vi "子VI-查看某框.vi"(0 "输入框号（默认值0为整张图）":dbl format="%#_13g", 1 "框组":T3(array[cluster]), 2 "临界Z值":i32, 3 "反射图原始路径":path, 4 "临界面积百分比值":dbl, 5 "预先配置的灰度阈值":dbl, 6 "穿透图原始路径":path, 7 "部位信息":string[](array[string])=["", "34.500000", "32.500000", "1121", "34", "54.955926", "分层类", "不合格", ""], 12 "产品规格":cluster{"产品长度（周长）（mm）":dbl, "产品宽度（母线长）（mm）":dbl}) -> (14 "弥散类检测结果":string[][](table), 19 "分层类检测结果":string[][](table))   [LabVIEW 2018]
uses:
  <vilib>/vision/NI_Vision_Development_Module.lvlib
panel:
  in  "返回主界面":bool caption="辅助定性分析"
  in  "格式字符串 3":string="%f"
  in  "分隔符（'\\'代码显示） 2":string="\t"
  out "弥散和分层临界灰度值":i64
  out "弥散缺陷个数":i32
  out "分层缺陷个数":i32
  out "合格？ 弥散类":string="fencengThreshold"
  out "合格？分层类":string="fencengThreshold"
  in  "Tab Control":T1
  out "穿透ROI":T2(plugin-control)
  out "Threshold Image":T2(plugin-control)
  out "?":T2(plugin-control)
  out "?":T2(plugin-control)
  out "Threshold Image":T2(plugin-control)
  out "Threshold Image":T2(plugin-control)
  out "弥散测量结果":dbl[][](array[numeric]) format="%.2f"
  out "?":string
  out "面积 (pixels)":i32
  in  "格式字符串 2":string="%f"
  in  "分隔符（'\\'代码显示）":string="\t"
  out "分层测量结果":dbl[][](array[numeric]) format="%.2f"
  out "缺陷初步分类的临界值":sgl format="%#.3f"
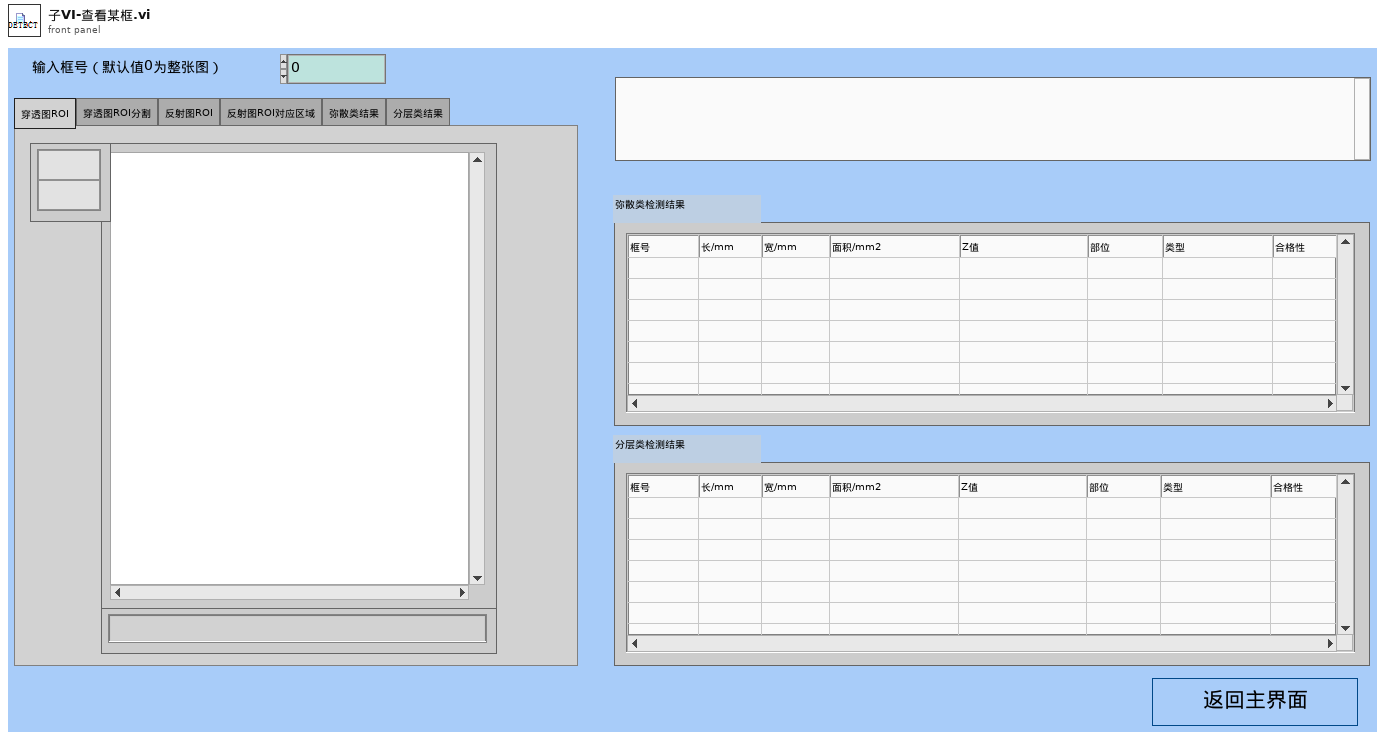
[diagram p1: front panel]
types:
  T1 = typedef "控件 1.ctl" = enum32{"穿透图ROI", "穿透图ROI分割", "反射图ROI", "反射图ROI对应区域", "弥散类结果", "分层类结果"}
  T2 = typedef "IMAQ Image.ctl" = refnum<image>
  T3 = cluster{"Global Rectangle":i32[], "Contours":cluster{"Contour Type":u32, "ROI Type":u32, "Points":i32[]}[]}[]
  T4 = cluster{"Zoom Tool":bool, "Selection Tool":bool, "Pan Tool":bool, "Point Tool":bool, "Line Tool":bool, "Rectangle Tool":bool, "Rotated Rectangle Tool":bool, "Polyline Tool":bool, "Polygon Tool":bool, "Freehand Tool":bool, "Closed Freehand Tool":bool, "Ellipse Tool":bool, "Annulus Tool":bool}
  T5 = typedef "Image Type" = u32
  T6 = typedef "Particle Parameters" = i32
  T7 = cluster{"Measurement Parameter":T6, "Range Lower Value":dbl, "Range Upper Value":dbl, "Range":bool, "Measurement Type":bool}[]
  T8 = cluster{"Global Rectangle":i32[], "Contours":cluster{"Contour Type":u32, "ROI Type":u32, "Points":i32[]}[]}
  T9 = cluster{"histogram":u32[], "Minimal Value":sgl, "Maximal Value":sgl, "Starting Value":sgl, "Interval Width":sgl, "Mean Value":sgl, "Standard  Variation":sgl, "Area (pixels)":i32}
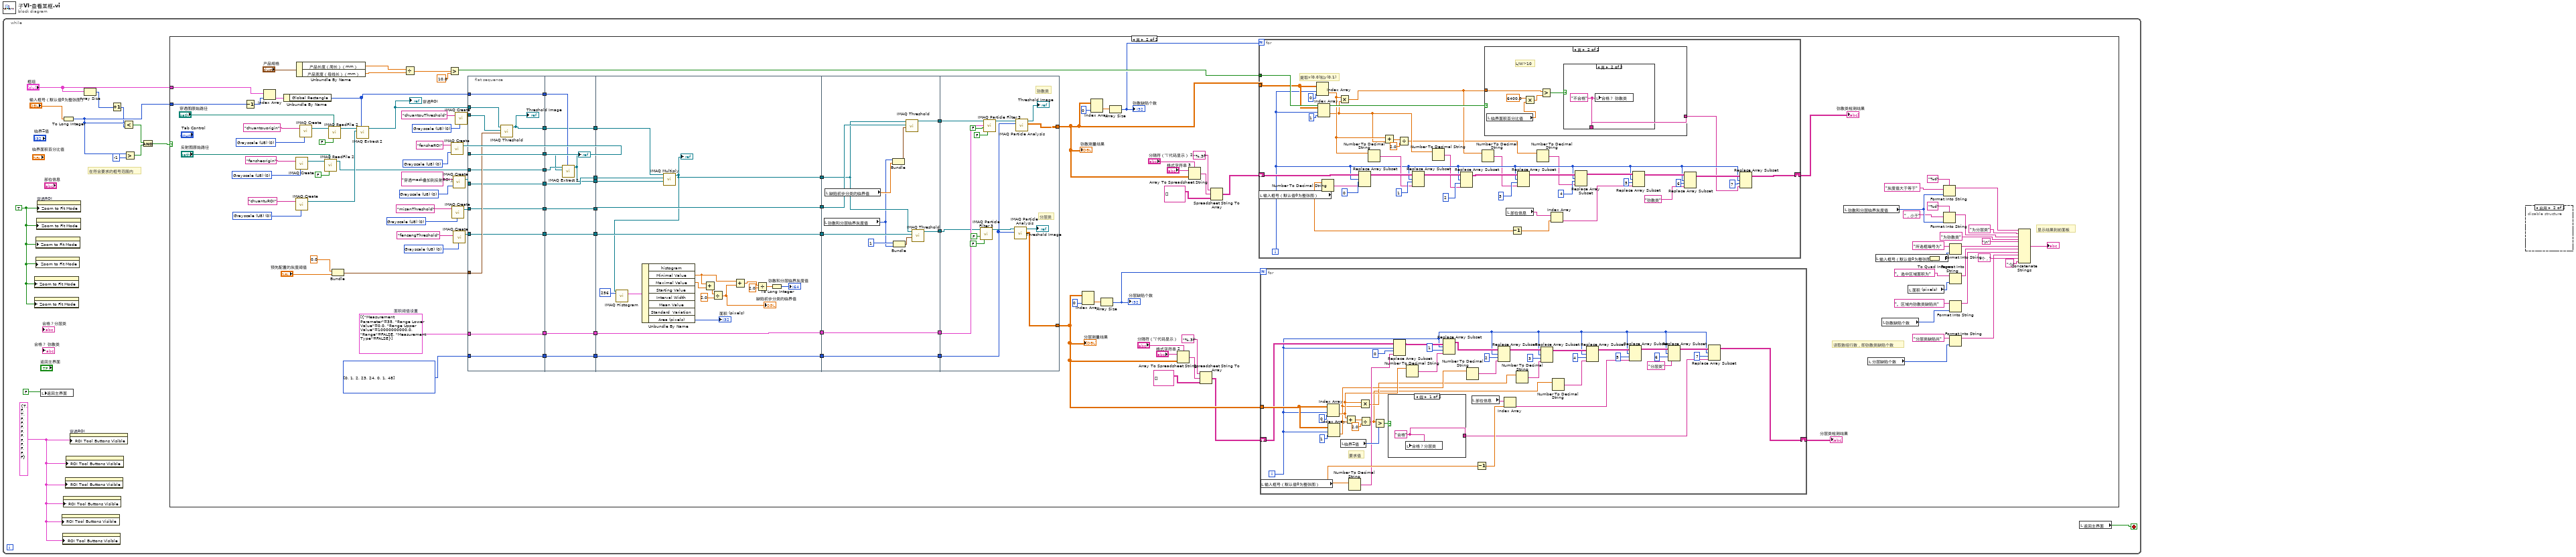
[diagram p0: block diagram]
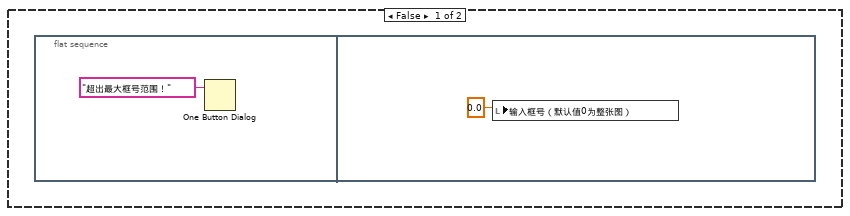
[diagram p2: hidden frame]
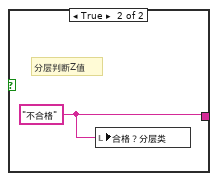
[diagram p3: hidden frame]
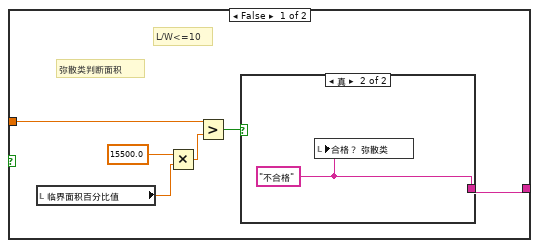
[diagram p4: hidden frame]
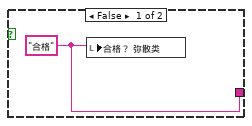
[diagram p5: hidden frame]
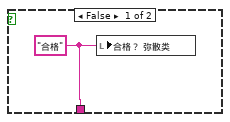
[diagram p6: hidden frame]
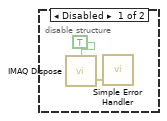
[diagram p7: hidden frame]
diagram:
  n1 = while {
    stop <- w5 stop-if-true
    w3 = T4 {"Zoom Tool"=TRUE, "Selection Tool"=FALSE, "Pan Tool"=TRUE, "Point Tool"=FALSE, "Line Tool"=FALSE, "Rectangle Tool"=FALSE, "Rotated Rectangle Tool"=FALSE, "Polyline Tool"=FALSE, "Polygon Tool"=FALSE, "Freehand Tool"=FALSE, "Closed Freehand Tool"=FALSE, "Ellipse Tool"=FALSE, "Annulus Tool"=FALSE} ("ROI Tool Buttons Visible:All Elements")
    w13 = TRUE ("Zoom to Fit Mode")
    # "在符合要求的框号范围内"
    n2 = property class="ImageControl"("Zoom to Fit Mode"=w13) -> ()  [unwired: 2 in, 2 out]
    n3 = property class="ImageControl"("Zoom to Fit Mode"=w13) -> ()  [unwired: 2 in, 2 out]
    n4 = property class="ImageControl"("Zoom to Fit Mode"=w13) -> ()  [unwired: 2 in, 2 out]
    n5 = property class="ImageControl"("Zoom to Fit Mode"=w13) -> ()  [unwired: 2 in, 2 out]
    n6 = property class="ImageControl"("Zoom to Fit Mode"=w13) -> ()  [unwired: 2 in, 2 out]
    n7 = property on="穿透ROI" class="ImageControl"("Zoom to Fit Mode"=w13) -> ()  [unwired: 2 in, 2 out]
    n8 = local write "返回主界面"(FALSE ("stop")) -> ()
    n9 = property class="ImageControl"("ROI Tool Buttons Visible"=w3) -> ()  [unwired: 2 in, 2 out]
    n10 = To Long Integer(number="输入框号（默认值0为整张图）") -> (32bit integer=w6:i32)
    n11 = property class="ImageControl"("ROI Tool Buttons Visible"=w3) -> ()  [unwired: 2 in, 2 out]
    n12 = property class="ImageControl"("ROI Tool Buttons Visible"=w3) -> ()  [unwired: 2 in, 2 out]
    n13 = property class="ImageControl"("ROI Tool Buttons Visible"=w3) -> ()  [unwired: 2 in, 2 out]
    n14 = property class="ImageControl"("ROI Tool Buttons Visible"=w3) -> ()  [unwired: 2 in, 2 out]
    n15 = property on="穿透ROI" class="ImageControl"("ROI Tool Buttons Visible"=w3) -> ()  [unwired: 2 in, 2 out]
    n16 = Array Size(array="框组") -> (size(s)=w2:i32)
    n17 = Increment(x=w2) -> (x+1=w1:i32)
    n18 = Less?(x=w6, y=w1) -> (x < y?=w11:bool)
    n19 = Greater?(x=w6, y=-1) -> (0:w10:bool)
    n20 = And(x=w11, y=w10) -> (x .and. y?=w4:bool)
    n21 = case shown="真" w4 {
      tunnel: "框组" -> [_ w17]
      tunnel: w6 -> [_ w16]
      frame False {
        n22 = flat-sequence {
          frame #0 {
            n23 = One Button Dialog(message="超出最大框号范围！" ("消息")) -> ()  [unwired: 1 in, 1 out]
          }
          frame #1 {
            n24 = local write "输入框号（默认值0为整张图）"(0.0 ("框号")) -> ()
          }
        }
      }
      frame True {
        w80 = T5 0 items=["Grayscale (U8)", "Grayscale (I16)", "Grayscale (SGL)", "Complex (CSG)", "RGB (U32)", "HSL (U32)", "RGB (U64)", "Grayscale (U16)"] ("Image Type")
        w81 = T5 0 items=["Grayscale (U8)", "Grayscale (I16)", "Grayscale (SGL)", "Complex (CSG)", "RGB (U32)", "HSL (U32)", "RGB (U64)", "Grayscale (U16)"] ("Image Type")
        w82 = T5 0 items=["Grayscale (U8)", "Grayscale (I16)", "Grayscale (SGL)", "Complex (CSG)", "RGB (U32)", "HSL (U32)", "RGB (U64)", "Grayscale (U16)"] ("Image Type")
        w86 = T5 0 items=["Grayscale (U8)", "Grayscale (I16)", "Grayscale (SGL)", "Complex (CSG)", "RGB (U32)", "HSL (U32)", "RGB (U64)", "Grayscale (U16)"] ("Image Type")
        w90 = T5 0 items=["Grayscale (U8)", "Grayscale (I16)", "Grayscale (SGL)", "Complex (CSG)", "RGB (U32)", "HSL (U32)", "RGB (U64)", "Grayscale (U16)"] ("Image Type")
        w64 = i32[] [0, 1, 2, 23, 24, 0, 1, 48] items=["Bounding Rect Width", "Bounding Rect Height", "Area"] ("Pixel Measurements")
        w65 = T7 [{"Measurement Parameter"=35, "Range Lower Value"=0.0, "Range Upper Value"=10000000000.0, "Range"=FALSE, "Measurement Type"=FALSE}]  # 面积阈值设置
        w101 = T5 0 items=["Grayscale (U8)", "Grayscale (I16)", "Grayscale (SGL)", "Complex (CSG)", "RGB (U32)", "HSL (U32)", "RGB (U64)", "Grayscale (U16)"] ("Image Type")
        w74 = T5 0 items=["Grayscale (U8)", "Grayscale (I16)", "Grayscale (SGL)", "Complex (CSG)", "RGB (U32)", "HSL (U32)", "RGB (U64)", "Grayscale (U16)"] ("Image Type")
        w105 = T5 0 items=["Grayscale (U8)", "Grayscale (I16)", "Grayscale (SGL)", "Complex (CSG)", "RGB (U32)", "HSL (U32)", "RGB (U64)", "Grayscale (U16)"] ("Image Type")
        # "显示结果到前面板"
        # "读取数组行数，即弥散类缺陷个数"
        n25 = Decrement(x=w16) -> (x-1=w107:i32)
        n26 = Index Array(array=w17, index=w107) -> (element=w108:T8)
        n27 = Unbundle By Name(w108) -> ("Global Rectangle"=w73:i32[])
        n28 = call "IMAQ Create"("Image Name"="fansheorigin", "Image Type"=w86) -> ("New Image"=w85:T2)  [unwired: 3 in, 1 out]
        n29 = call "IMAQ Create"("Image Name"="chuantuROI", "Image Type"=w90) -> ("New Image"=w89:T2)  [unwired: 3 in, 1 out]
        n30 = Unbundle By Name("产品规格") -> ("产品长度（周长）（mm）"=w96:dbl, "产品宽度（母线长）（mm）"=w95:dbl)
        n31 = call "IMAQ Create"("Image Name"="chuantouorigin", "Image Type"=w105) -> ("New Image"=w92:T2)  [unwired: 3 in, 1 out]
        n32 = call "IMAQ ReadFile 2"("Use File Path Image Type"=FALSE, "File Path"="反射图原始路径", "Image"=w85) -> ("Image Out"=w69:T2)  [unwired: 4 in, 4 out]
        n33 = call "IMAQ ReadFile 2"("Use File Path Image Type"=FALSE, "File Path"="穿透图原始路径", "Image"=w92) -> ("Image Out"=w93:T2)  [unwired: 4 in, 4 out]
        n34 = Bundle(0.0, "预先配置的灰度阈值"="预先配置的灰度阈值") -> (w63:cluster{dbl, "预先配置的灰度阈值":dbl})  [unwired: 1 in]
        n35 = call "IMAQ Extract 2"("Optional Rectangle"=w73, "Image Dst"=w89, "Image Src"=w93) -> ("Image Dst Out"=w71:T2)  [unwired: 7 in, 1 out]
        "穿透ROI" <- w71
        n36 = Divide(x=w96, y=w95) -> (x/y=w99:dbl)
        n37 = Greater?(x=w99, y=10.0) -> (0:w48:bool)
        n38 = call "IMAQ Create"("Image Name"="fansheROI", "Image Type"=w74) -> ("New Image"=w70:T2)  [unwired: 3 in, 1 out]
        n39 = call "IMAQ Create"("Image Name"="misanThreshold", "Image Type"=w80) -> ("New Image"=w67:T2)  [unwired: 3 in, 1 out]
        n40 = call "IMAQ Create"("Image Name"="穿透mask叠加到反射ROI上", "Image Type"=w101) -> ("New Image"=w68:T2)  [unwired: 3 in, 1 out]
        n41 = call "IMAQ Create"("Image Name"="fencengThreshold", "Image Type"=w81) -> ("New Image"=w66:T2)  [unwired: 3 in, 1 out]
        n42 = call "IMAQ Create"("Image Name"="chuantouThreshold", "Image Type"=w82) -> ("New Image"=w72:T2)  [unwired: 3 in, 1 out]
        n43 = flat-sequence {
          tunnel: w73 -> [w189]
          tunnel: w72 -> [w188]
          tunnel: w71 -> [w187]
          tunnel: w63 -> [w186]
          tunnel: w70 -> [w185]
          tunnel: w69 -> [w184]
          tunnel: [w189] -> w135
          tunnel: [w185] -> w134
          tunnel: [w184] -> w133
          tunnel: [w183] -> w132
          tunnel: w68 -> [w183]
          tunnel: [w182] -> w131
          tunnel: w67 -> [w181]
          tunnel: [w181] -> w130
          tunnel: [w180] -> w129
          tunnel: w66 -> [w180]
          tunnel: [w179] -> w128
          tunnel: w65 -> [w179]
          tunnel: [w178] -> w127
          tunnel: w64 -> [w178]
          tunnel: w135 -> [w199]
          tunnel: w134 -> [w190]
          tunnel: w133 -> [w191]
          tunnel: w132 -> [w198]
          tunnel: [w198] -> w126
          tunnel: [w197] -> w125
          tunnel: w131 -> [w197]
          tunnel: [w196] -> w124
          tunnel: w130 -> [w195]
          tunnel: [w195] -> w123
          tunnel: w129 -> [w194]
          tunnel: [w194] -> w122
          tunnel: w128 -> [w193]
          tunnel: [w193] -> w121
          tunnel: w127 -> [w192]
          tunnel: [w192] -> w120
          tunnel: w126 -> [w219]
          tunnel: w125 -> [w218]
          tunnel: w124 -> [w217]
          tunnel: [w216] -> w119
          tunnel: w123 -> [w216]
          tunnel: w122 -> [w215]
          tunnel: [w215] -> w118
          tunnel: [w210] -> w117
          tunnel: w121 -> [w209]
          tunnel: [w209] -> w116
          tunnel: w120 -> [w208]
          tunnel: [w208] -> w115
          tunnel: w119 -> [w231]
          tunnel: w118 -> [w230]
          tunnel: w117 -> [w229]
          tunnel: [w228] -> w114
          tunnel: [w227] -> w113
          tunnel: w116 -> [w226]
          tunnel: [w226] -> w112
          tunnel: w115 -> [w225]
          tunnel: [w225] -> w111
          tunnel: [w236] -> w45
          tunnel: [w240] -> w52
          tunnel: w114 -> [w233]
          tunnel: w113 -> [w232]
          tunnel: w112 -> [w238]
          tunnel: w111 -> [w237]
          frame #0 {
            n44 = call "IMAQ Threshold"("Range"=w186, "Image Dst"=w188, "Image Src"=w187) -> ("Image Dst Out"=w182:T2)  [unwired: 3 in, 5 out]
            "Threshold Image" <- w182
          }
          frame #1 {
            n45 = call "IMAQ Extract 2"("Optional Rectangle"=w199, "Image Dst"=w190, "Image Src"=w191) -> ("Image Dst Out"=w196:T2)  [unwired: 7 in, 1 out]
            "?" <- w196
          }
          frame #2 {
            n46 = call "IMAQ Multiply"("Image Src A"=w218, "Image Dst"=w219, "Image Src B"=w217) -> ("Image Dst Out"=w210:T2)  [unwired: 4 in, 1 out]
            "?" <- w210
            n47 = call "IMAQ Histogram"("Number of Classes"=256, "Image"=w210) -> ("Histogram Report"=w213:T9)  [unwired: 8 in, 1 out]
            n48 = Unbundle By Name(w213) -> ("Minimal Value"=w202:sgl, "Maximal Value"=w204:sgl, "Area (pixels)"=→"面积 (pixels)":i32)  [unwired: 5 out]
            n49 = Add(x=w202, y=w204) -> (x+y=w203:sgl)
            n50 = Divide(x=w203, y=sgl 2.0) -> (x/y=w201:sgl)
            "缺陷初步分类的临界值" <- w201
            n51 = Add(x=w202, y=w201) -> (x+y=w200:sgl)
            n52 = Divide(x=w200, y=sgl 2.0) -> (x/y=w205:sgl)
            n53 = To Long Integer(number=w205) -> (32bit integer=→"弥散和分层临界灰度值":i32)
          }
          frame #3 {
            n54 = local read "弥散和分层临界灰度值"() -> (w221:i64)
            n55 = local read "缺陷初步分类的临界值"() -> (w223:sgl)
            n56 = Bundle("弥散和分层临界灰度值"=w221, "缺陷初步分类的临界值"=w223) -> (w224:cluster{"弥散和分层临界灰度值":i64, "缺陷初步分类的临界值":sgl})  [unwired: 1 in]
            n57 = Bundle(1, "弥散和分层临界灰度值"=w221) -> (w220:cluster{i32, "弥散和分层临界灰度值":i64})  [unwired: 1 in]
            n58 = call "IMAQ Threshold"("Range"=w224, "Image Dst"=w231, "Image Src"=w229) -> ("Image Dst Out"=w227:T2)  [unwired: 3 in, 5 out]
            n59 = call "IMAQ Threshold"("Range"=w220, "Image Dst"=w230, "Image Src"=w229) -> ("Image Dst Out"=w228:T2)  [unwired: 3 in, 5 out]
          }
          frame #4 {
            # "分层类"
            # "弥散类"
            n60 = call "IMAQ Particle Filter 3"("Image Src"=w233, "Keep/Remove Particles (F)"=FALSE, "Reject Border? (F)"=FALSE) -> ("Image Dst Out"=w242:T2)  [unwired: 10 in, 2 out]
            n61 = call "IMAQ Particle Filter 3"("Image Src"=w232, "Selection Values"=w238, "Keep/Remove Particles (F)"=FALSE, "Reject Border? (F)"=FALSE) -> ("Image Dst Out"=w244:T2)  [unwired: 9 in, 2 out]
            n62 = call "IMAQ Particle Analysis"("Pixel Measurements"=w237, "Image"=w242) -> ("Particle Measurements (Pixels)"=w240:dbl[][], "Image Out (duplicate)"=→"Threshold Image":T2)  [unwired: 4 in, 4 out]
            n63 = call "IMAQ Particle Analysis"("Pixel Measurements"=w237, "Image"=w244) -> ("Particle Measurements (Pixels)"=w236:dbl[][], "Image Out (duplicate)"=→"Threshold Image":T2)  [unwired: 4 in, 4 out]
          }
        }
        n64 = Index Array(array=w52, index (col)=0 ("禁用的索引 (列)")) -> (element=w79:dbl[])  [unwired: 1 in]
        n65 = Index Array(array=w45, index (col)=0 ("禁用的索引 (列)")) -> (element=w77:dbl[])  [unwired: 1 in]
        n66 = Array Size(array=w79) -> (size(s)=w50:i32)
        "分层缺陷个数" <- w50
        n67 = Array Size(array=w77) -> (size(s)=w47:i32)
        "弥散缺陷个数" <- w47
        n68 = Array To Spreadsheet String(delimiter (Tab)="分隔符（'\\'代码显示）", array=w52, 3:"格式字符串 2") -> (spreadsheet string=w60:string)
        n69 = Array To Spreadsheet String(delimiter (Tab)="分隔符（'\\'代码显示） 2", array=w45, 3:"格式字符串 3") -> (spreadsheet string=w55:string)
        n70 = Spreadsheet String To Array(format string="%.3f", spreadsheet string=w60, array type (2D Dbl)=string[][] [] ("Array")) -> (array=w51:string[][])  [unwired: 1 in]
        n71 = Spreadsheet String To Array(format string="%.3f", spreadsheet string=w55, array type (2D Dbl)=string[][] [] ("Array")) -> (array=w46:string[][])  [unwired: 1 in]
        n72 = for {
          N: w47 -> [_]
          tunnel: w48 -> [w284]
          tunnel: w45 -> [w283]
          shift-right: [w263] -> w44
          shift-left: w46 -> [w271]
          i -> [w261]
          # "提取x(0,0)和y(0,1)"
          n73 = local read "输入框号（默认值0为整张图）"() -> (w249:dbl)
          n74 = Index Array(array=w283, index (row)=w261, index (col)=0 ("禁用的索引 (列)")) -> (element=w255:dbl)
          n75 = Index Array(array=w283, index (row)=w261, index (col)=1 ("禁用的索引 (列)")) -> (element=w254:dbl)
          n76 = Number To Decimal String(number=w249) -> (decimal integer string=w272:string)  [unwired: 1 in]
          n77 = Multiply(x=w255, y=w254) -> (x*y=w259:dbl)
          n78 = Replace Array Subset(array=w271, new element=w272, index (row)=w261, index (col)=0 ("索引 (列)")) -> (w270:string[][])
          n79 = Number To Decimal String(number=w255) -> (decimal integer string=w262:string)  [unwired: 1 in]
          n80 = Add(x=w255, y=w254) -> (x+y=w257:dbl)
          n81 = Divide(x=w257, y=2.0) -> (x/y=w253:dbl)
          n82 = Replace Array Subset(array=w270, new element=w262, index (row)=w261, index (col)=1 ("索引 (列)")) -> (w269:string[][])
          n83 = Number To Decimal String(number=w254) -> (decimal integer string=w260:string)  [unwired: 1 in]
          n84 = Replace Array Subset(array=w269, new element=w260, index (row)=w261, index (col)=2 ("索引 (列)")) -> (w268:string[][])
          n85 = Number To Decimal String(number=w259) -> (decimal integer string=w258:string)  [unwired: 1 in]
          n86 = case shown="真" w284 {
            tunnel: w259 -> [w290 w298]
            tunnel: [w288 w296] -> w246
            frame False {
              # "弥散类判断面积"
              # "L/W<=10"
              n87 = local read "临界面积百分比值"() -> (w286:dbl)
              n88 = Multiply(x=15500.0, y=w286) -> (x*y=w285:dbl)
              n89 = Greater?(x=w290, y=w285) -> (0:w289:bool)
              n90 = case shown="真" w289 {
                tunnel: [w291 w292] -> w288
                frame False {
                  w291 = "合格" ("合格？")
                  n91 = local write "合格？ 弥散类"(w291) -> ()
                }
                frame True {
                  w292 = "不合格" ("合格？")
                  n92 = local write "合格？ 弥散类"(w292) -> ()
                }
              }
            }
            frame True {
              # "L/W>10"
              n93 = local read "临界面积百分比值"() -> (w293:dbl)
              n94 = Multiply(x=6400.0, y=w293) -> (x*y=w295:dbl)
              n95 = Greater?(x=w298, y=w295) -> (0:w297:bool)
              n96 = case shown="真" w297 {
                tunnel: [w299 w300] -> w296
                frame False {
                  w299 = "合格" ("合格？")
                  n97 = local write "合格？ 弥散类"(w299) -> ()
                }
                frame True {
                  w300 = "不合格" ("合格？")
                  n98 = local write "合格？ 弥散类"(w300) -> ()
                }
              }
            }
          }
          n99 = local read "部位信息"() -> (w251:string[])
          n100 = Decrement(x=w249) -> (x-1=w250:dbl)
          n101 = Replace Array Subset(array=w268, new element=w258, index (row)=w261, index (col)=3 ("索引 (列)")) -> (w267:string[][])
          n102 = Number To Decimal String(number=w253) -> (decimal integer string=w252:string)  [unwired: 1 in]
          n103 = Index Array(array=w251, index=w250) -> (element=w248:string)
          n104 = Replace Array Subset(array=w267, new element=w252, index (row)=w261, index (col)=4 ("索引 (列)")) -> (w266:string[][])
          n105 = Replace Array Subset(array=w266, new element=w248, index (row)=w261, index (col)=5 ("索引 (列)")) -> (w265:string[][])
          n106 = Replace Array Subset(array=w265, new element="弥散类" ("新元素/子数组"), index (row)=w261, index (col)=6 ("索引 (列)")) -> (w264:string[][])
          n107 = Replace Array Subset(array=w264, new element=w246, index (row)=w261, index (col)=7 ("索引 (列)")) -> (w263:string[][])
        }
        "弥散类检测结果" <- w44
        n108 = for {
          N: w50 -> [_]
          tunnel: w52 -> [w167]
          shift-right: [w145] -> w49
          shift-left: w51 -> [w156]
          i -> [w140]
          # "要求值"
          n109 = local read "输入框号（默认值0为整张图）"() -> (w165:dbl)
          n110 = Index Array(array=w167, index (row)=w140, index (col)=0 ("禁用的索引 (列)")) -> (element=w144:dbl)
          n111 = Index Array(array=w167, index (row)=w140, index (col)=1 ("禁用的索引 (列)")) -> (element=w143:dbl)
          n112 = local read "临界Z值"() -> (w173:i32)
          n113 = Add(x=w144, y=w143) -> (x+y=w174:dbl)
          n114 = Number To Decimal String(number=w165) -> (decimal integer string=w157:string)  [unwired: 1 in]
          n115 = Multiply(x=w144, y=w143) -> (x*y=w142:dbl)
          n116 = Divide(x=w174, y=2.0) -> (x/y=w139:dbl)
          n117 = Greater?(x=w139, y=w173) -> (0:w175:bool)
          n118 = case shown="假" w175 {
            tunnel: [w176 w177] -> w136
            frame False {
              w176 = "合格" ("合格？")
              n119 = local write "合格？分层类"(w176) -> ()
            }
            frame True {
              w177 = "不合格" ("合格？")
              # "分层判断Z值"
              n120 = local write "合格？分层类"(w177) -> ()
            }
          }
          n121 = Replace Array Subset(array=w156, new element=w157, index (row)=w140, index (col)=0 ("索引 (列)")) -> (w155:string[][])
          n122 = Number To Decimal String(number=w144) -> (decimal integer string=w154:string)  [unwired: 1 in]
          n123 = Replace Array Subset(array=w155, new element=w154, index (row)=w140, index (col)=1 ("索引 (列)")) -> (w152:string[][])
          n124 = Number To Decimal String(number=w143) -> (decimal integer string=w153:string)  [unwired: 1 in]
          n125 = local read "部位信息"() -> (w169:string[])
          n126 = Decrement(x=w165) -> (x-1=w168:dbl)
          n127 = Replace Array Subset(array=w152, new element=w153, index (row)=w140, index (col)=2 ("索引 (列)")) -> (w151:string[][])
          n128 = Index Array(array=w169, index=w168) -> (element=w138:string)
          n129 = Number To Decimal String(number=w142) -> (decimal integer string=w150:string)  [unwired: 1 in]
          n130 = Replace Array Subset(array=w151, new element=w150, index (row)=w140, index (col)=3 ("索引 (列)")) -> (w149:string[][])
          n131 = Number To Decimal String(number=w139) -> (decimal integer string=w141:string)  [unwired: 1 in]
          n132 = Replace Array Subset(array=w149, new element=w141, index (row)=w140, index (col)=4 ("索引 (列)")) -> (w148:string[][])
          n133 = Replace Array Subset(array=w148, new element=w138, index (row)=w140, index (col)=5 ("索引 (列)")) -> (w147:string[][])
          n134 = Replace Array Subset(array=w147, new element="分层类" ("新元素/子数组"), index (row)=w140, index (col)=6 ("索引 (列)")) -> (w146:string[][])
          n135 = Replace Array Subset(array=w146, new element=w136, index (row)=w140, index (col)=7 ("索引 (列)")) -> (w145:string[][])
        }
        "分层类检测结果" <- w49
        n136 = local read "弥散和分层临界灰度值"() -> (w43:i64)
        n137 = local read "分层缺陷个数"() -> (w19:i32)
        n138 = local read "输入框号（默认值0为整张图）"() -> (w34:dbl)
        n139 = local read "弥散缺陷个数"() -> (w18:i32)
        n140 = local read "面积 (pixels)"() -> (w37:i32)
        n141 = To Quad Integer(1:w34) -> (0:w35:i64)
        n142 = Format Into String(format string="%d" ("格式字符串"), initial string="灰度值大于等于" ("初始字符串"), w43) -> (resulting string=w39:string)  [unwired: 1 in, 1 out]
        n143 = Format Into String(format string="%d" ("格式字符串"), initial string="，小于" ("初始字符串"), w43) -> (resulting string=w38:string)  [unwired: 1 in, 1 out]
        n144 = Format Into String(initial string="所选框编号为" ("初始字符串"), w35) -> (resulting string=w33:string)  [unwired: 2 in, 1 out]
        n145 = Format Into String(initial string="。选中区域面积为" ("字符串"), w37) -> (resulting string=w40:string)  [unwired: 2 in, 1 out]
        n146 = Format Into String(initial string="。区域内弥散类缺陷共" ("初始字符串"), w18) -> (resulting string=w41:string)  [unwired: 2 in, 1 out]
        n147 = Format Into String(initial string="分层类缺陷共" ("初始字符串"), w19) -> (resulting string=w42:string)  [unwired: 2 in, 1 out]
        n148 = Concatenate Strings(w39, "为分层类" ("初始字符串"), w38, "为弥散类" ("初始字符串"), "\n", w33, w40, w41, "个，" ("字符串"), w42, "个" ("字符串")) -> (→"?":string)
        "分层测量结果" <- w52
        "弥散测量结果" <- w45
      }
    }
    n149 = local read "返回主界面"() -> (w5:bool)
  }
  n150 = disable-structure shown="启用" {
    frame Disabled {
      n151 = call "IMAQ Dispose"("All Images? (No)"=TRUE) -> ("error out"=w302:errorcluster)  [unwired: 5 in]
      n152 = call <vilib>:"Simple Error Handler.vi"("error in (no error)"=w302) -> ()  [unwired: 4 in, 5 out]
    }
    frame Enabled {
    }
  }
